vi "Analysis.Calculate Yield Item.vi"(10 "Pass Cnt":i32, 11 "Total Cnt":i32) -> (3 "Yield":T1)   [LabVIEW 2024]
uses:
  Analysis.Yield Info, Item.ctl
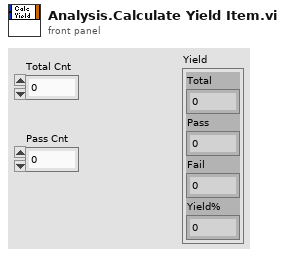
[diagram p1: front panel]
types:
  T1 = typedef "Analysis.Yield Info, Item.ctl" = cluster{"Total":i32, "Pass":i32, "Fail":i32, "Yield%":dbl}
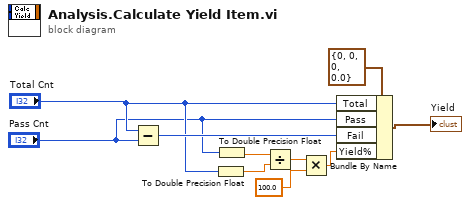
[diagram p0: block diagram]
diagram:
  n1 = Subtract(x="Total Cnt", y="Pass Cnt") -> (x-y=w9:i32)
  n2 = To Double Precision Float(number="Total Cnt") -> (double precision float=w5:dbl)
  n3 = To Double Precision Float(number="Pass Cnt") -> (double precision float=w6:dbl)
  n4 = Divide(x=w6, y=w5) -> (x/y=w4:dbl)
  n5 = Multiply(x=w4, y=100.0) -> (x*y=w3:dbl)
  n6 = Bundle By Name(cluster=T1 {"Total"=0, "Pass"=0, "Fail"=0, "Yield%"=0.0} ("All"), "Total"="Total Cnt", "Pass"="Pass Cnt", "Fail"=w9, "Yield%"=w3) -> (→"Yield":T1)
